vi "Synthetic_Jet_Measurement.vi"() -> (5 "Plug in titles":string[](array[string]), 7 "Plug in values":string[](array[string]))   [LabVIEW 2011]
uses:
  Controls/SJ_Channels.ctl
  Controls/SJ_Data_Cluster.ctl
  <vilib>/Analysis/2dsp.llb/Integral Method.ctl
  Globals/Meas_global.vi
  Globals/Plug_in_data_global.vi
  <vilib>/Analysis/5stat.llb/RMS (DBL).vi
  <vilib>/Analysis/8numeric.llb/1D Numeric Integration.vi
  Utilities/Get_Circ_Area.vi
  <vilib>/Analysis/baseanly.llb/Quick Scale 1D.vi
  <vilib>/Analysis/1siggen.llb/Ramp Pattern by Samples.vi
  <vilib>/Analysis/NI_AALBase.lvlib
  <vilib>/Analysis/NI_AALPro.lvlib
panel:
  out "Jet ID":string="A"
  out "Disc ID":i32
  out "RMS Power 2 _W_":dbl
  out "RMS Input Voltage _V_":dbl format="%0.2f"
  out "Jet Efficiency":dbl
  out "Int Power _W_":dbl
  out "Phase Average?":bool
  out "Samps per cyle":i32
  out "Formation Criteria":dbl
  out "Jet Formation":bool
  out "Strouhal Number":dbl
  out "Stokes Number":dbl
  out "nu":dbl=1.55e-05
  out "Omega":dbl=1200.0
  out "Reynolds Number":dbl
  out "Charicteristic Velocity m_s":dbl
  out "Stroke Length _m_":dbl
  out "DL:Frequency":dbl=2.802671520827615
  out "Cavity:Helmholtz:Hz":dbl=428.16291209383184
  out "DL:Radius":dbl
  out "DL:Streamwise:Position":dbl=5.0
  out "LEM Velocity _ms_":dbl[](array[numeric])=[3.7049856348371377, 3.4607988115264297, 3.0653584733968287, 2.5359472607578692, 1.895702983998723, 1.1726073902466658, 0.3982632267462864, -0.3934869508418966, -1.1680398605184126, -1.8915438234131698, -2.5323782445904723, -3.062535584780142, -3.458845424238726, -3.7039871212762807, -3.787246807411894, -3.7049856348371377, -3.4607988115264297, -3.0653584733968295, -2.5359472607578692, -1.8957029839987247, -1.172607390246666, -0.3982632267462887, 0.3934869508418962, 1.1680398605184101, 1.8915438234131694, 2.53237824459047, 3.0625355847801417, 3.4588454242387248, 3.7039871212762803, 3.7872468074118935]
  out "LEM Max Velocity _ms_":dbl=3.7872475686779676
  out "LEM Phase Velocity _deg_":dbl=-258.0363282123533
  out "Phase Power _deg_":dbl=-1216.295394809798
  out "Phase Current _deg_":dbl=114.2968039724566
  out "RV Phase Pressure _deg_":dbl
  out "Phase Pressure _deg_":dbl=-169.14507601114087
  out "Phase Displ _deg_":dbl=-40.709415815185025
  out "Phase Velocity _deg_":dbl=373.1272896341652
  out "Phase Input Voltage _deg_":dbl=8.606071626556414
  out "Phase Angle _deg_":dbl[](array[numeric])=[0.0, 12.0, 24.0, 36.0, 48.0, 60.0, 72.0, 84.0, 96.0, 108.0, 120.0, 132.0, 144.0, 156.0, 168.0, 180.0, 192.0, 204.0, 216.0, 228.0, 240.0, 252.0, 264.0, 276.0, 288.0, 300.0, 312.0, 324.0, 336.0, 348.0]
  out "Max Power _W_":dbl=0.09567394666235574 format="%0.2f"
  out "Amplitude (V)":dbl=70.0
  out "Frequency (Hz)":dbl=1200.0
  out "AS Freq":dbl=36036.04
  out "Output Data Names":string[](array[string])=["Max Pressure _Pa_", "Max Velocity m_s", "Max Current _A_", "Max Displacement _m_", "Phase Displ _deg_", "Phase Pressure _deg_", "Phase Velocity _deg_", "Phase Current _deg_", "Phase Input Voltage _deg_", "LEM Max Velocity _ms_", "LEM Phase Velocity _deg_"]
  out "Current _A_":dbl[](array[numeric])=[0.007871578951352444, 0.008266417140890889, 0.00849968074403876, 0.008455354076272185, 0.007734598407207069, 0.006567672714377243, 0.00502412226480415, 0.003160545427498193, 0.0011561900642313688, -0.0008322812950871137, -0.0026496409136783387, -0.004250177970402979, -0.0056599044207173484, -0.006974613805967722, -0.007544462997563997, -0.008243629249997945, -0.008448348909812501, -0.008596065082556333, -0.008270248882544743, -0.007591372292965107, -0.0065346555924612445, -0.005182607825984795, -0.003607407527949277, -0.0016626720392260718, 0.00036386353784322137, 0.0021437834956932957, 0.003704399543557329, 0.005128068807114345, 0.006438338773620389, 0.007353635511234548]
  out "Power_W_":dbl[](array[numeric])=[-0.043363451952469156, -0.1045787042911587, -0.16349661489678932, -0.21135096948039916, -0.2294893577920496, -0.21702510361561647, -0.17587031608696657, -0.11191242161210375, -0.03966959410717387, 0.026383849953920794, 0.07342545396353153, 0.09567394666235574, 0.0925358489049179, 0.06622858320017053, 0.01657193795313242, -0.042740863570043953, -0.10421979243576313, -0.16261661392816973, -0.2041915474460092, -0.22315321729709184, -0.2143088761872366, -0.18014115682356102, -0.12703551569073906, -0.05674338994484436, 0.011476164341731257, 0.059131235834024416, 0.08299512964242624, 0.08340916969883025, 0.06053396412209597, 0.01568890358261011]
  out "RV Pressure _V_":dbl[](array[numeric])=[-14.369666524328046, -57.77058962565634, -87.07652966541758, -117.51006835010423, -142.3114261743131, -158.09199483911908, -155.83679754926837, -151.8902022920296, -142.3114261743131, -120.32906496241762, -88.20412831034297, -49.31359978871612, -12.114469234477319, 29.02544421285115, 67.35217341201532, 101.7323073539407, 128.78305010385122, 147.3826153809706, 157.5310031852989, 162.59938472331393, 149.63781267082135, 136.11244129586606, 102.29610667640338, 72.99016663664214, 42.55081558780641, -5.354689729074237, -48.18600114379076, -84.25753305310417, -116.38246970517886, -138.36483091707433, -158.65579416158175, -165.41557366698484, -160.34719212896982, -149.0712056797162, -122.58426225226835, -92.71452289004439, -56.642990980730964, -17.188663136641456, 24.515049633149694, 61.15038086492581, 97.22191277423924, 132.1658460386273, 151.3292106382094, 160.34418743346322, 160.34418743346322, 155.27580589544817, 136.67624061832876, 106.80650125610484, 74.67575223988108, 33.5358387925526, -1.9718937942981463, -42.553820283313044, -85.38513169802953, -116.38246970517886, -141.74762685185044, -159.78339280650712, -164.28797502205947, -162.03859009635784, -141.18382752938774, -123.71186089719372, -94.40592085743245, -59.46198759304437, -20.007659748954865, 21.70186538498539, 58.3313842526124, 92.14771887207513, 124.27846788829885, 149.63781267082135, 160.34418743346322, 156.9672038628362, 155.27580589544817, 141.75043452049292, 110.18348482673184, 77.49474885219449, 41.987016265343726, 0.2833034955525799, -41.42622163838768, -76.37015490277572, -109.62269019977577, -131.59923904752216, -159.21959348404445, -167.67077095683558, -160.9109914514325, -151.8902022920296, -125.96705818704444, -102.29329900776088, -63.96656980859674, -33.53303112391013, 16.627671482821253, 53.82680203706004, 93.27531751700047, 122.58706992091082, 148.51021402589598, 158.65860183022428, 155.27580589544817, 156.9672038628362, 142.30842147880648, 120.3318726310601, 80.31374546450789, 48.18880881243323, 10.425878935731753, -34.6606297688355, -76.37015490277572, -108.49509155485042, -133.85443633737287, -151.8902022920296, -162.03859009635784, -164.28797502205947, -154.709198904343, -135.54583430476092, -104.54849629761163, -71.85976032307427, -32.96923180144745, 7.0430830009556615, 52.135404069672006, 85.95173868913471, 118.64047466367205, 142.30842147880648, 157.5310031852989, 159.78038811100052, 158.09480250776156, 142.30842147880648, 123.71466856583618, 86.5155380115974, 49.316407457358586, 13.244875548045162, -27.33705094096973, -69.04076371076087, -103.42089765268625, -130.4716404025968, -151.8902022920296, -160.34719212896982, -162.60238941882054, -154.14539958188033, -135.54583430476092, -104.54849629761163, -71.85976032307427, -36.91582705868622, 4.793698075254034, 51.007805424746635, 81.44134410943326, 115.82147805135864, 140.62283587556755, 154.1482072505228, 160.9079867559259, 156.40340454037351, 145.69121741358256, 120.89567195352278, 93.27531751700047, 54.95440068198541]
  out "Displacement _m_":dbl[](array[numeric])=[-2.6563452608725367e-05, -3.3033094590941884e-05, -3.489470009695634e-05, -3.608459414033635e-05, -3.599336290251176e-05, -3.300271431749379e-05, -3.056117109155232e-05, -2.2626856342716373e-05, -1.762170629215838e-05, -1.0755312405507711e-05, -5.5370483534114006e-06, -2.8768068802271785e-07, 4.656075893275746e-06, 8.287603580077764e-06, 1.4940431377787088e-05, 1.9792866303780654e-05, 2.4126214474223672e-05, 2.519431617137013e-05, 2.644560368400959e-05, 2.7208727219429685e-05, 2.372973382223118e-05, 2.04641256790127e-05, 1.719906004067715e-05, 1.3689415117589209e-05, 8.043566800208257e-06, 4.4422385518931854e-06, -1.2338996214552368e-06, -5.841845680176716e-06, -1.1396101089811283e-05, -1.6401251140369278e-05]
  out "Input Voltage _V_":dbl[](array[numeric])=[-5.5088632433799996, -12.651031578584, -19.235618350895997, -24.9961110527, -29.670494279084004, -33.04444558276, -35.005182361704, -35.409211536216006, -34.310616683552006, -31.700640287920002, -27.711473499856005, -22.510574222680006, -16.349366000988, -9.495663135284, -2.196569584672, 5.184714435096, 12.336113665324001, 18.917564300223997, 24.689891482827996, 29.395636083331993, 32.795741589576, 34.758786092276, 35.215182844328, 34.127830748423996, 31.539748142271996, 27.582652797175996, 22.404475723135995, 16.265220463328, 9.402109185388, 2.133489422836]
  out "Pressure _Pa_":dbl[](array[numeric])=[-27.3956675953706, 95.65286233449294, 217.28142105099454, 325.3916285730047, 412.49320713856633, 477.62511872885386, 518.8812420389512, 544.5955786383588, 546.2858417945154, 525.7943338813993, 485.98446016799124, 431.53940396868336, 357.29264741860004, 257.81676584697294, 146.44897730607346, 25.39291194062997, -95.29994862668336, -216.63005998968256, -325.4638615668826, -412.65459893301875, -477.423305725176, -519.6780076017092, -543.7330519967387, -544.6659346048561, -524.568602441649, -487.2326508157636, -435.0203186855821, -361.9795522274816, -267.2741357434412, -152.01151538796677]
  out "Zeros":dbl[](array[numeric])=[1.4978743085562871, 0.2341330189017041, -0.35175473981443495, 0.0022887999999999997, -3.0068544366899315, 2.8293]
  out "Velocity m_s":dbl[](array[numeric])=[-0.006589971422005106, -0.006419643065741468, -0.009111611844261746, -0.006030326884042168, -0.004272653157727323, -0.0068849933436421745, -0.010636233235274354, -0.0035467148583991693, -0.008496862890472292, -0.005357351691532665, -0.007065956289182962, -0.006648911559621155, -0.005058171342073957, -0.008830133605031026, -0.0038751674420970687, -0.005274584307176274, 0.000979796600094568, -0.005616008146962059, -0.00729733372181674, 0.0005036149760482819, -0.004633370846616606, -0.007598533001820504, -0.005354959759266961, -0.003855515705978843, -0.005082756078867318, -0.0008163141834672163, -0.007346968606858383, -0.00413574997102441, -0.00277648312445221, -0.00052352239052674]
  out "Max Current _A_":dbl=0.00849968074403876 format="%e"
  out "RMS Dispacement _m_":dbl=2.25005755896471e-05 format="%0.2f"
  out "RMS Velocity m_s":dbl=0.014914535983039488 format="%0.2f"
  out "RMS Current _A_":dbl=0.006206722435388947 format="%0.2f"
  out "RV RMS Pressure _V_":dbl format="%0.2f"
  out "RMS Pressure _Pa_":dbl=395.7699897259115 format="%0.2f"
  out "RMS Power _W_":dbl=0.13002833315099252 format="%0.2f"
  out "Max Displacement _m_":dbl=2.7208727219429685e-05 format="%e"
  out "Max Pressure _Pa_":dbl=546.2858417945154 format="%0.2f"
  out "RV Max Pressure _V_":dbl format="%0.2f"
  out "Max Velocity m_s":dbl=0.000979796600094568
  out "Current Plot":cluster{dbl[], dbl[]}[](graph)=[{[0.0, 12.0, 24.0, 36.0, 48.0, 60.0, 72.0, 84.0, 96.0, 108.0, 120.0, 132.0, 144.0, 156.0, 168.0, 180.0, 192.0, 204.0, 216.0, 228.0, 240.0, 252.0, 264.0, 276.0, 288.0, 300.0, 312.0, 324.0, 336.0, 348.0], [-0.15557712257291065, -0.35728080433659803, -0.5432376920119246, -0.705921142218441, -0.8379315153272326, -0.9332160799164545, -0.9885897155857659, -1.0, -0.9689743203815658, -0.8952653536353687, -0.7826063416157439, -0.6357265029653804, -0.4617263500562873, -0.2681692905127802, -0.06203384626131485, 0.1464227586596542, 0.34838713233438734, 0.5342554516040381, 0.697273122209331, 0.8301691793748806, 0.926192371045399, 0.9816311796924717, 0.9945203893712923, 0.9638122191316959, 0.8907215601232357, 0.7789682853842954, 0.632730149899583, 0.45934997583022086, 0.26552721106968635, 0.060252384345070756]}, {[0.0, 12.0, 24.0, 36.0, 48.0, 60.0, 72.0, 84.0, 96.0, 108.0, 120.0, 132.0, 144.0, 156.0, 168.0, 180.0, 192.0, 204.0, 216.0, 228.0, 240.0, 252.0, 264.0, 276.0, 288.0, 300.0, 312.0, 324.0, 336.0, 348.0], [0.915718863893427, 0.9616512975995976, 0.9887873884629885, 0.9836307653638304, 0.8997836024883751, 0.7640324556993839, 0.5844676856855597, 0.36767351074525567, 0.13450224644966696, -0.09682119517406056, -0.3082388148799797, -0.49443296782707047, -0.6584296845544803, -0.8113728478069623, -0.8776647134598465, -0.9590003298982027, -0.9828158382556238, -1.0, -0.962097052909388, -0.8831217795651628, -0.7601914980520298, -0.6029046751288172, -0.41965800552972216, -0.19342245821289428, 0.04232908131205239, 0.24939125926856856, 0.4309413095387709, 0.5965600257634787, 0.7489867412341333, 0.855465313560387]}]
  in  "Menu Ring":u16(ring) items=["Max Pressure _Pa_", "RMS Pressure _Pa_", "Phase Pressure _deg_", "Max Current _A_", "RMS Current _A_", "Phase Current _deg_", "Max Power _W_", "RMS Power _W_", "RMS Power 2 _W_", "Int Power _W_", "Phase Power _deg_"]
  out "Pressure v Frequency":cluster{dbl[], dbl[]}(graph)
  out "Pressure Plot":cluster{dbl[], dbl[]}[](graph)=[{[0.0, 12.0, 24.0, 36.0, 48.0, 60.0, 72.0, 84.0, 96.0, 108.0, 120.0, 132.0, 144.0, 156.0, 168.0, 180.0, 192.0, 204.0, 216.0, 228.0, 240.0, 252.0, 264.0, 276.0, 288.0, 300.0, 312.0, 324.0, 336.0, 348.0], [-0.15557712257291065, -0.35728080433659803, -0.5432376920119246, -0.705921142218441, -0.8379315153272326, -0.9332160799164545, -0.9885897155857659, -1.0, -0.9689743203815658, -0.8952653536353687, -0.7826063416157439, -0.6357265029653804, -0.4617263500562873, -0.2681692905127802, -0.06203384626131485, 0.1464227586596542, 0.34838713233438734, 0.5342554516040381, 0.697273122209331, 0.8301691793748806, 0.926192371045399, 0.9816311796924717, 0.9945203893712923, 0.9638122191316959, 0.8907215601232357, 0.7789682853842954, 0.632730149899583, 0.45934997583022086, 0.26552721106968635, 0.060252384345070756]}, {[0.0, 12.0, 24.0, 36.0, 48.0, 60.0, 72.0, 84.0, 96.0, 108.0, 120.0, 132.0, 144.0, 156.0, 168.0, 180.0, 192.0, 204.0, 216.0, 228.0, 240.0, 252.0, 264.0, 276.0, 288.0, 300.0, 312.0, 324.0, 336.0, 348.0], [-0.05014896140338823, 0.1750967259562854, 0.39774309423293575, 0.5956435325215701, 0.7550867615085017, 0.8743135592895557, 0.9498346878887768, 0.9969058997564276, 1.0, 0.9624894032658751, 0.8896156974736197, 0.7899516534258018, 0.6540397353973438, 0.47194480640402603, 0.2680812243366908, 0.0464828300459258, -0.17445070206035157, -0.39655074947222896, -0.5957757581594167, -0.7553821962097238, -0.87394413180629, -0.9512932019153176, -0.9953270072140422, -0.9970346894139926, -0.9602456485390019, -0.8919005647578826, -0.7963236192550169, -0.6626193185574809, -0.4892569334498257, -0.2782636922981901]}]
  out "Displacement Plot":cluster{dbl[], dbl[]}[](graph)=[{[0.0, 12.0, 24.0, 36.0, 48.0, 60.0, 72.0, 84.0, 96.0, 108.0, 120.0, 132.0, 144.0, 156.0, 168.0, 180.0, 192.0, 204.0, 216.0, 228.0, 240.0, 252.0, 264.0, 276.0, 288.0, 300.0, 312.0, 324.0, 336.0, 348.0], [-0.15557712257291065, -0.35728080433659803, -0.5432376920119246, -0.705921142218441, -0.8379315153272326, -0.9332160799164545, -0.9885897155857659, -1.0, -0.9689743203815658, -0.8952653536353687, -0.7826063416157439, -0.6357265029653804, -0.4617263500562873, -0.2681692905127802, -0.06203384626131485, 0.1464227586596542, 0.34838713233438734, 0.5342554516040381, 0.697273122209331, 0.8301691793748806, 0.926192371045399, 0.9816311796924717, 0.9945203893712923, 0.9638122191316959, 0.8907215601232357, 0.7789682853842954, 0.632730149899583, 0.45934997583022086, 0.26552721106968635, 0.060252384345070756]}, {[0.0, 12.0, 24.0, 36.0, 48.0, 60.0, 72.0, 84.0, 96.0, 108.0, 120.0, 132.0, 144.0, 156.0, 168.0, 180.0, 192.0, 204.0, 216.0, 228.0, 240.0, 252.0, 264.0, 276.0, 288.0, 300.0, 312.0, 324.0, 336.0, 348.0], [-0.7361438653132033, -0.9154348379941063, -0.9670248738630008, -1.0, -0.997471739948916, -0.9145929198799676, -0.8469312685822951, -0.6270503211070746, -0.48834431180314575, -0.2980582894650082, -0.15344632481876624, -0.00797239638899362, 0.12903223672595104, 0.2296715198692966, 0.4140390583217413, 0.5485129256769343, 0.668601519540294, 0.6982014560947281, 0.7328779584207091, 0.7540261396210363, 0.6576139870090829, 0.5671153068654675, 0.47663166097388826, 0.3793700731217815, 0.22290861216080401, 0.12310623571424707, -0.03419463765219268, -0.16189306875552578, -0.3158162468307329, -0.45452225613466185]}]
  out "Velocity Plot":cluster{dbl[], dbl[]}[](graph)=[{[0.0, 12.0, 24.0, 36.0, 48.0, 60.0, 72.0, 84.0, 96.0, 108.0, 120.0, 132.0, 144.0, 156.0, 168.0, 180.0, 192.0, 204.0, 216.0, 228.0, 240.0, 252.0, 264.0, 276.0, 288.0, 300.0, 312.0, 324.0, 336.0, 348.0], [-0.15557712257291065, -0.35728080433659803, -0.5432376920119246, -0.705921142218441, -0.8379315153272326, -0.9332160799164545, -0.9885897155857659, -1.0, -0.9689743203815658, -0.8952653536353687, -0.7826063416157439, -0.6357265029653804, -0.4617263500562873, -0.2681692905127802, -0.06203384626131485, 0.1464227586596542, 0.34838713233438734, 0.5342554516040381, 0.697273122209331, 0.8301691793748806, 0.926192371045399, 0.9816311796924717, 0.9945203893712923, 0.9638122191316959, 0.8907215601232357, 0.7789682853842954, 0.632730149899583, 0.45934997583022086, 0.26552721106968635, 0.060252384345070756]}, {[0.0, 12.0, 24.0, 36.0, 48.0, 60.0, 72.0, 84.0, 96.0, 108.0, 120.0, 132.0, 144.0, 156.0, 168.0, 180.0, 192.0, 204.0, 216.0, 228.0, 240.0, 252.0, 264.0, 276.0, 288.0, 300.0, 312.0, 324.0, 336.0, 348.0], [-0.0017400427690923374, -0.0016950685794170583, -0.002405866928563968, -0.0015922719565676093, -0.001128168660507009, -0.0018179415532591603, -0.002808434141249664, -0.0009364889690996669, -0.002243546122698781, -0.0014145768585897204, -0.0018657237429983216, -0.001755605561963586, -0.0013355800662831847, -0.0023315442732039188, -0.0010232149208002786, -0.001392722622896813, 0.00025870946624789303, -0.0014828735576385352, -0.0019268175782828233, 0.00013297653986074366, -0.0012234140213805954, -0.002006347457194939, -0.0014139452830977239, -0.0010180259967302217, -0.001342071519849202, -0.00021554290622666447, -0.0019399233745421283, -0.001092020188103525, -0.0007331138596561618, -0.00013823297428152076]}, {[0.0, 12.0, 24.0, 36.0, 48.0, 60.0, 72.0, 84.0, 96.0, 108.0, 120.0, 132.0, 144.0, 156.0, 168.0, 180.0, 192.0, 204.0, 216.0, 228.0, 240.0, 252.0, 264.0, 276.0, 288.0, 300.0, 312.0, 324.0, 336.0, 348.0], [0.9782794265180274, 0.9138033477917035, 0.8093896778519208, 0.6696017951074252, 0.5005491008108334, 0.3096200089077361, 0.10515903689372944, -0.10389788964157722, -0.3084139798421589, -0.49945089918916635, -0.6686594176102914, -0.8086443108979737, -0.9132875674934984, -0.9780157749495838, -1.0, -0.9782794265180274, -0.9138033477917035, -0.8093896778519211, -0.6696017951074252, -0.5005491008108338, -0.30962000890773617, -0.10515903689373006, 0.10389788964157712, 0.3084139798421583, 0.4994508991891662, 0.6686594176102908, 0.8086443108979736, 0.9132875674934979, 0.9780157749495837, 0.9999999999999999]}]
  out "Amplitude String":string="3.5000"
  out "Frequency String":string="1200"
  # "You Must have selected the \"Save Data\" option on the \nMeasurement Program for this vi to work correctly"
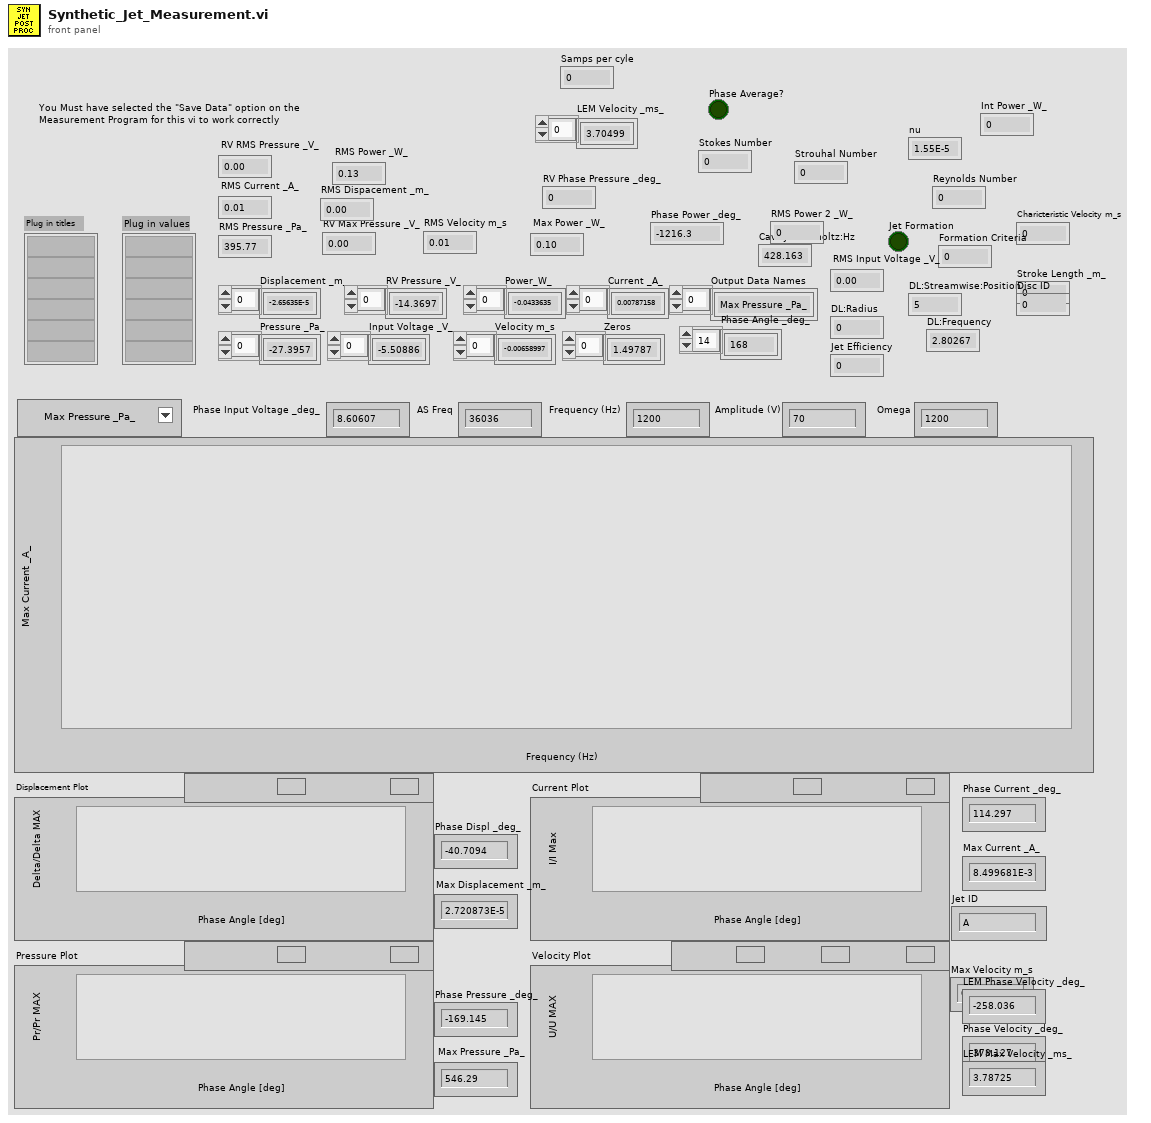
[diagram p1: front panel]
types:
  T1 = typedef "SJ_Channels.ctl" = string[]
  T2 = typedef "Analysis_info_cluster.ctl" = cluster{"Colour":u32, "Inst type":T3, "Inst name":string, "Symbol":string, "Code name":string, "Extra Info":string, "Inst Array":T4, "Extra Titles":string[], "Extra Values":string[], "Eng Values":dbl[], "Time (ms)":dbl[], "Voltage":dbl[], "U":dbl, "u^2":dbl, "u^3":dbl, "u^4":dbl, "Skew_u":dbl, "Kurt_u":dbl, "Sd Error in Mean":dbl, "% u'/U":dbl, "X":dbl, "Y":dbl, "Z":dbl, "Spectra":T5, "Autocorrelation":T5, "Timescale integral to 25%":dbl, "Sd Error in Variance":dbl, "Calib File":path, "Calib Constants":dbl[], "Histogram":T5, "Output Position":bool, "Full Stats":bool, "Weighting":dbl[], "Av Sampling Rate":dbl, "Av No of Samples":dbl, "Total Meas Time (s)":dbl}
  T3 = typedef "Inst_type.ctl" = enum16{"Propeller anemometer", "Raw voltage", "Pressure Transducer", "Pitot-static tube", "Preston tube", "Hot wire", "Cross wire 1", "Cross wire 2", "Generic Linear", "Generic Polynomial", "Generic BackPoly", "Fast FID", "Thermocouple", "Cold wire", "Pulsed Wire", "LDA Vel", "LDA Tran time", "LDA Arr time"}
  T4 = typedef "Instrument_Array.ctl" = enum16{"PWA", "LDA", "Analogue"}
  T5 = typedef "XY_Plot_Cluster.ctl" = cluster{"First Name":string, "Second Name":string, "X axis name":string, "Y axis name":string, "X array":dbl[], "Y array":dbl[]}
  T6 = typedef "Post_Process.ctl" = enum16{"Take New Data", "Post Process Raw Data File"}
  T7 = typedef "SJ_Data_Cluster.ctl" = cluster{"Do":dbl, "Dc":dbl, "Ho":dbl, "Hc":dbl, "K":dbl, "beta":dbl, "Vc":dbl, "Vo":dbl}
  T8 = cluster{"R":dbl, "Mair":dbl, "T":dbl, "Patmos":dbl, "gamma":dbl}
  T9 = typedef "NI_AALPro.lvlib/Integral Method.ctl" = i32
  T10 = cluster{"Ramp Pattern":dbl[], "Y[i]=X[i]/Max|X|":dbl[]}
  T11 = cluster{"Ramp Pattern":dbl[], "Y[i]=X[i]/Max|X|":dbl[]}[]
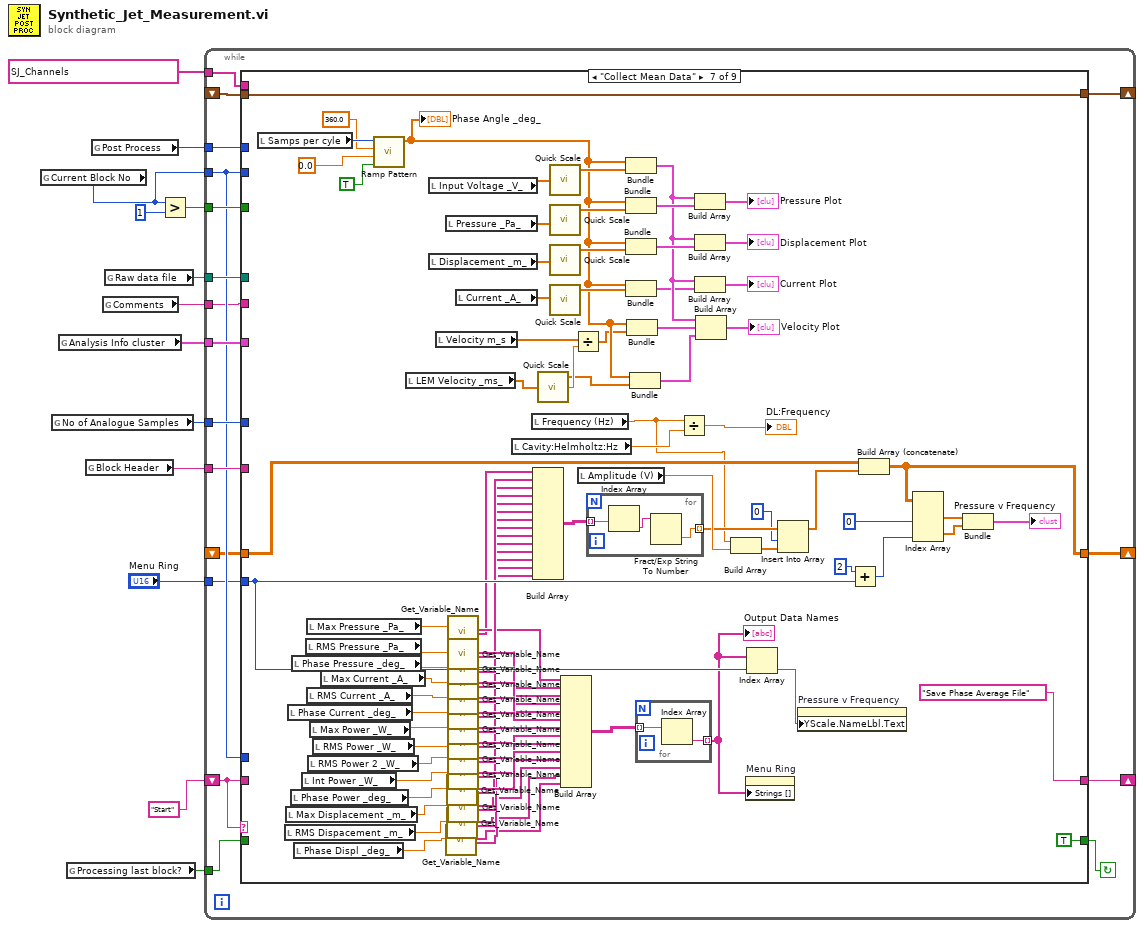
[diagram p0: block diagram]
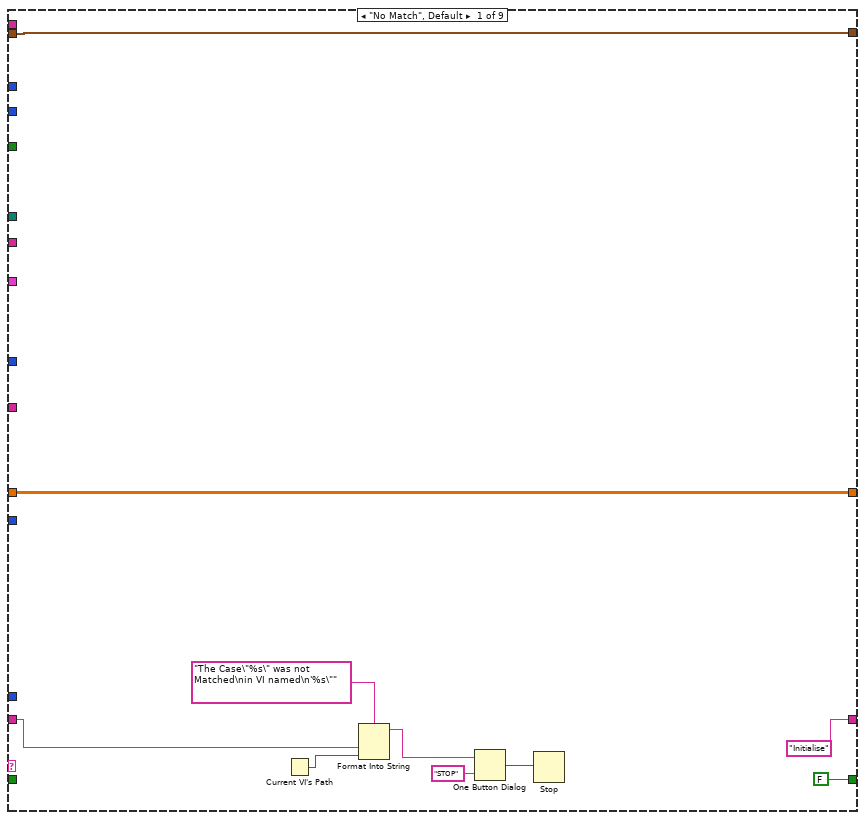
[diagram p2: hidden frame]
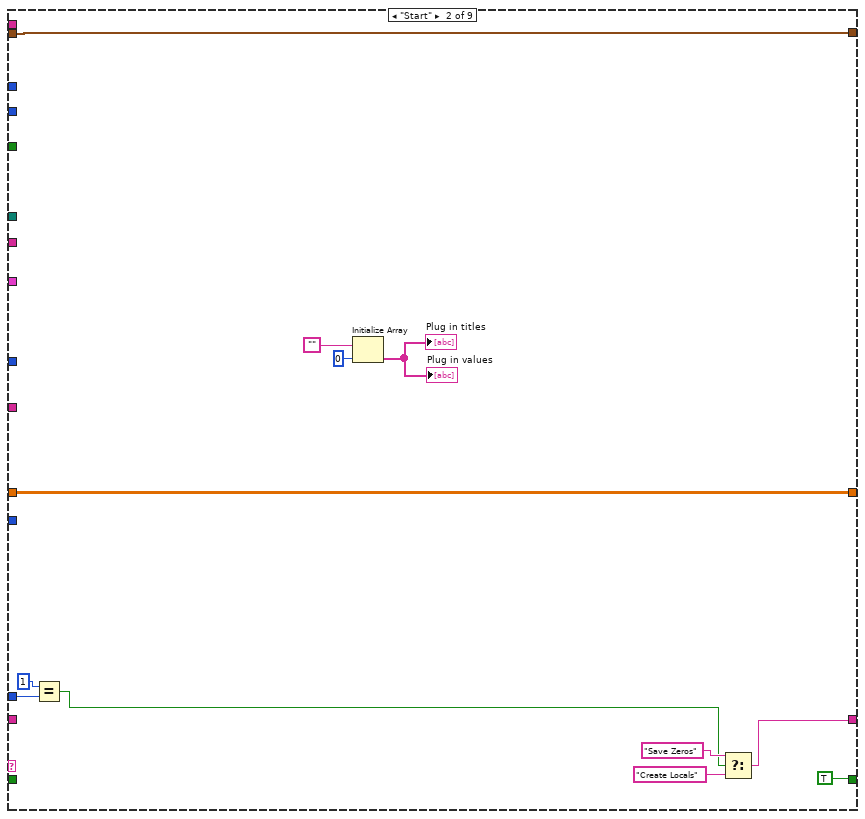
[diagram p3: hidden frame]
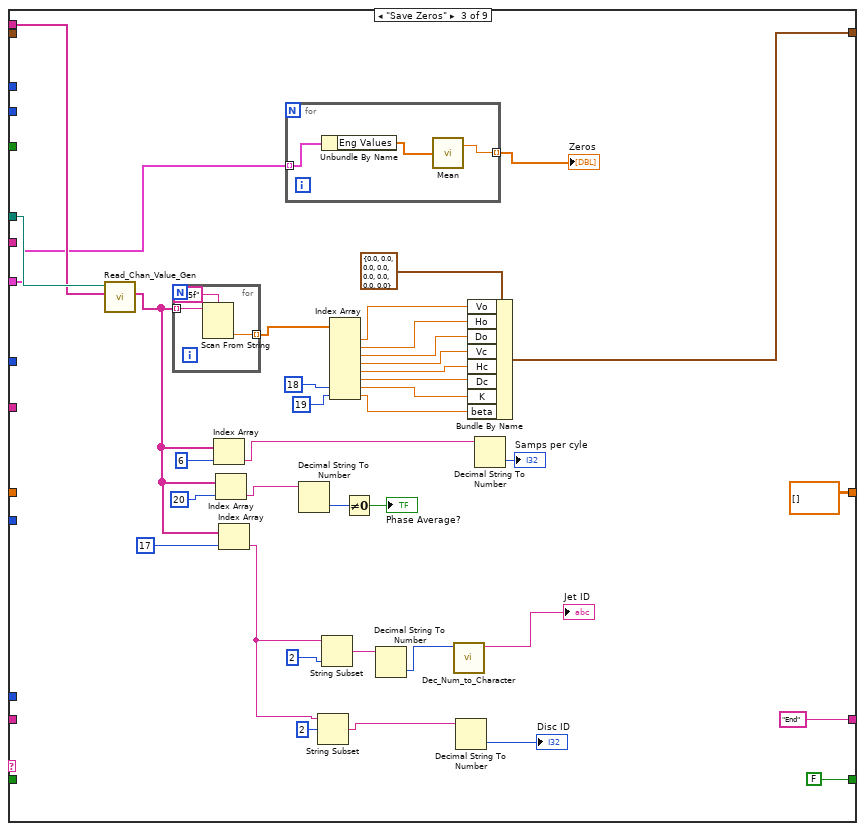
[diagram p4: hidden frame]
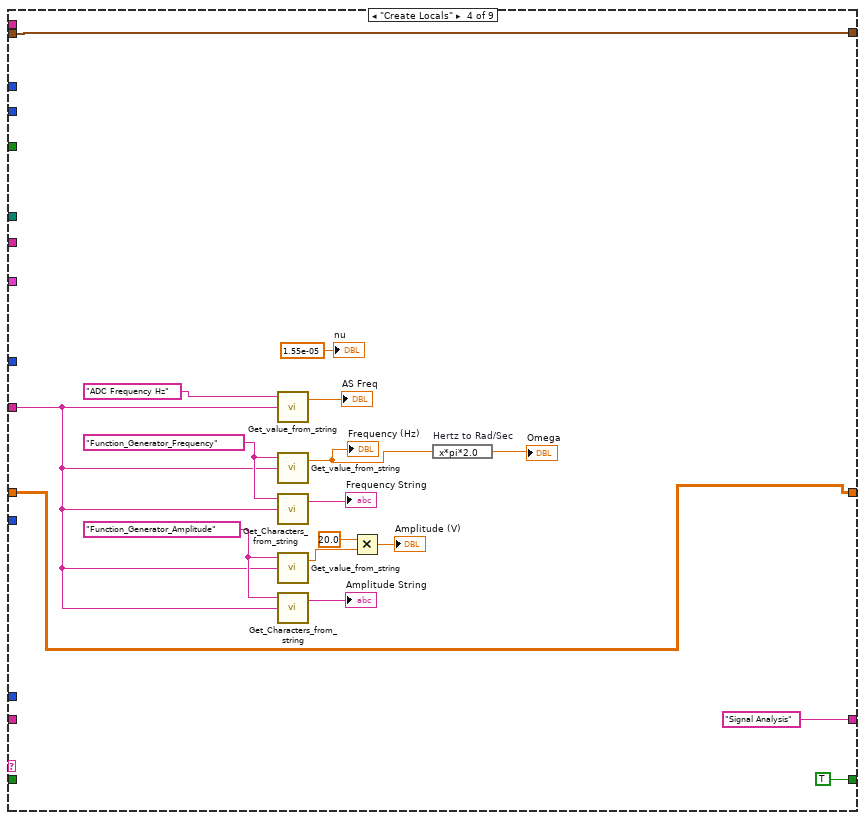
[diagram p5: hidden frame]
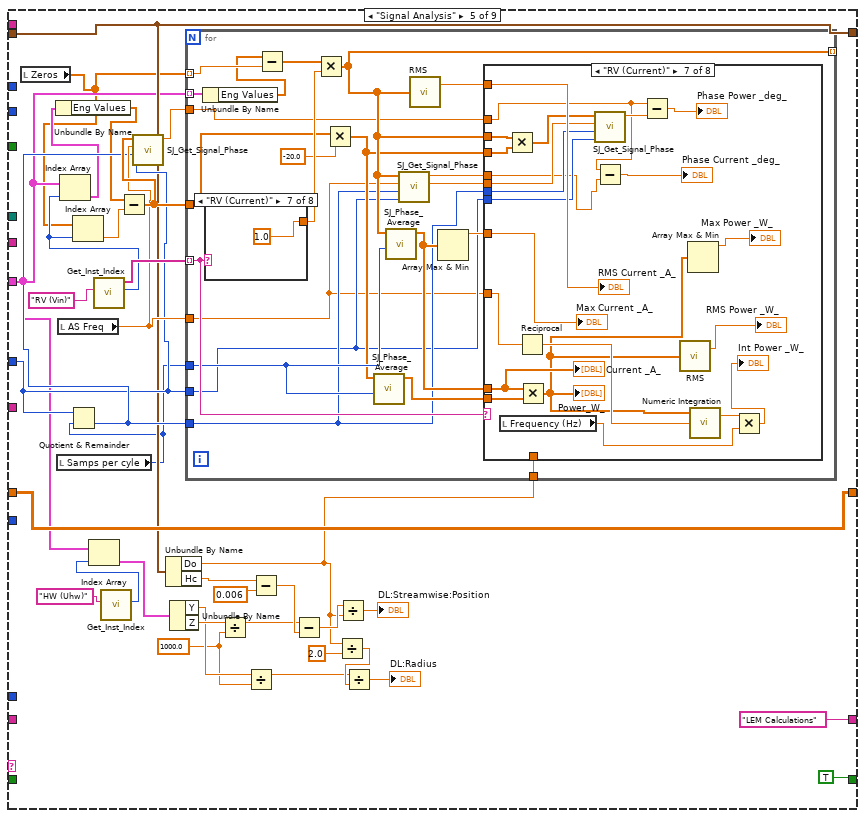
[diagram p6: hidden frame]
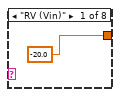
[diagram p7: hidden frame]
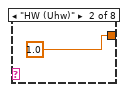
[diagram p8: hidden frame]
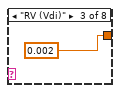
[diagram p9: hidden frame]
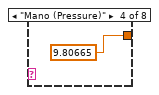
[diagram p10: hidden frame]
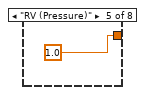
[diagram p11: hidden frame]
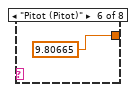
[diagram p12: hidden frame]
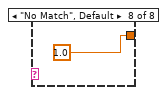
[diagram p13: hidden frame]
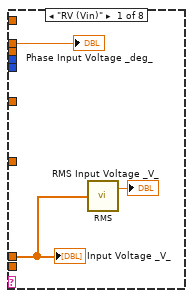
[diagram p14: hidden frame]
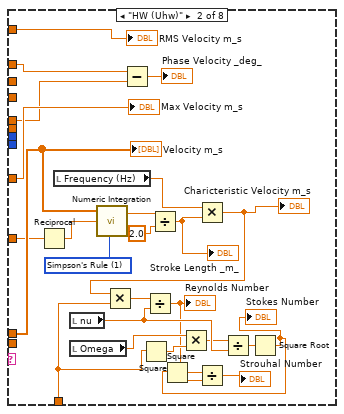
[diagram p15: hidden frame]
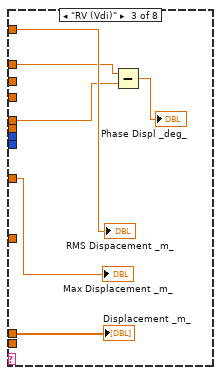
[diagram p16: hidden frame]
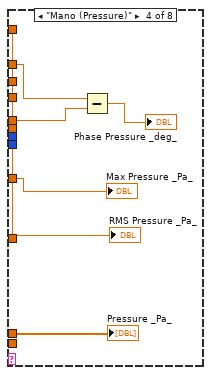
[diagram p17: hidden frame]
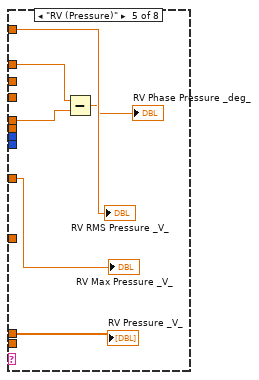
[diagram p18: hidden frame]
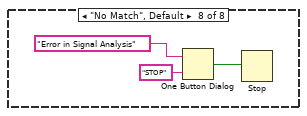
[diagram p20: hidden frame]
diagram:
  n1 = global read "Meas_global.vi" "Current Block No"() -> (w9:i32)
  n2 = global read "Meas_global.vi" "No of Analogue Samples"() -> (w6:i32)
  n3 = global read "Meas_global.vi" "Analysis Info cluster"() -> (w8:T2[])
  n4 = global read "Meas_global.vi" "Processing last block?"() -> (w5:bool)
  n5 = global read "Plug_in_data_global.vi" "Block Header"() -> (w7:string)
  n6 = global read "Meas_global.vi" "Post Process"() -> (w2:T6)
  n7 = global read "Meas_global.vi" "Comments"() -> (w4:string)
  n8 = global read "Meas_global.vi" "Raw data file"() -> (w12:path)
  n9 = Greater?(x=w9, y=1) -> (0:w10:bool)
  n10 = while {
    shift-left: "Start" -> [w31]
    shift-right: [w23] -> _
    tunnel: w12 -> [w30]
    tunnel: w10 -> [w29]
    tunnel: w9 -> [w24]
    tunnel: w8 -> [w28]
    tunnel: w7 -> [w27]
    tunnel: w6 -> [w26]
    tunnel: w5 -> [w25]
    shift-right: [w21] -> _
    shift-left: _ -> [w20]
    tunnel: w4 -> [w19]
    tunnel: "Menu Ring" -> [w18]
    tunnel: w2 -> [w17]
    shift-right: [w15] -> _
    shift-left: _ -> [w16]
    tunnel: T1 ["Synthetic_Jet:Orifice:Volume", "Synthetic_Jet:Orifice:Height", "Synthetic_Jet:Orifice:Diameter", "Synthetic_Jet:Cavity:Volume", "Synthetic_Jet:Cavity:Height", "Synthetic_Jet:Cavity:Diameter", "Synthetic_Jet:Samples:Per_Cycle", "Synthetic_Jet:Dwell:Time", "Synthetic_Jet:Minimum:Frequency", "Synthetic_Jet:Maximum:Frequency", "Synthetic_Jet:Minimum:Amplitude", "Synthetic_Jet:Maximum:Amplitude", "Synthetic_Jet:Amplitude:Delta", "Synthetic_Jet:Frequency:Delta", "Synthetic_Jet:Calibration:Velocity", "Synthetic_Jet:Calibration:Type", "Synthetic_Jet:Calibration:No_Of_Gens", "Synthetic_Jet:Identification:Number", "Synthetic_Jet:LEM_Pressure:Coefficient", "Synthetic_Jet:LEM_Added_Mass:Coefficient", "Synthetic_Jet:Phase:Average?", "Synthetic_Jet:Optimisation:Coefficient"] ("Synthetic Jet Specific Channels") -> [w14]
    stop <- w22 continue-if-true
    n11 = case shown="\"Collect Mean Data\"" w31 {
      tunnel: w31 -> [w37 _ _ _ _ _ _ _ _]
      tunnel: w30 -> [_ _ w84 _ _ w271 _ w468 w516]
      tunnel: w29 -> [_ _ _ _ _ _ _ _ _]
      tunnel: w24 -> [_ _ _ _ _ _ _ _ _]
      tunnel: w28 -> [_ _ w54 _ w116 _ _ _ _]
      tunnel: w27 -> [_ _ _ w108 _ _ _ _ _]
      tunnel: w26 -> [_ _ _ _ w138 _ _ _ _]
      tunnel: w25 -> [_ _ _ _ _ _ _ w395 _]
      tunnel: w24 -> [_ w50 _ _ _ _ _ _ _]
      tunnel: ["Initialise" w46 "End" ("t") "Signal Analysis" "LEM Calculations" "Collect Mean Data" "Save Phase Average File" "Save Mean Data" ("t") "End"] -> w23
      tunnel: [FALSE TRUE FALSE TRUE TRUE TRUE ("Processing last block?") TRUE ("Processing last block?") w395 FALSE ("Processing last block?")] -> w22
      tunnel: [w33 w44 dbl[][] [] w105 w144 w293 w379 w408 w558] -> w21
      tunnel: w20 -> [w33 w44 _ w105 w144 w293 w380 w408 w558]
      tunnel: w19 -> [_ _ _ _ _ _ _ w410 w532]
      tunnel: w18 -> [_ _ _ _ _ _ w354 _ _]
      tunnel: w17 -> [_ _ _ _ _ _ _ _ _]
      tunnel: w16 -> [w32 w42 _ w97 w133 w260 w316 w422 w557]
      tunnel: [w32 w42 w85 w97 w133 w260 w316 w422 w557] -> w15
      tunnel: w14 -> [_ _ w83 _ _ _ _ _ _]
      frame "No Match", Default {
        n12 = Current VI's Path() -> (path=w36:path)
        n13 = Format Into String(format string="The Case\"%s\" was not Matched\nin VI named\n'%s\"" ("Format String"), w37, w36) -> (resulting string=w40:string)  [unwired: 2 in, 1 out]
        n14 = One Button Dialog(message=w40, button name ("OK")="STOP") -> (true=w38:bool)
        n15 = Stop(stop? (T)=w38) -> ()
      }
      frame "Start" {
        n16 = Equal?(x=1, y=w50) -> (x = y?=w43:bool)
        n17 = Initialize Array("", 0) -> (→"Plug in values" →"Plug in titles":string[])
        n18 = Select(t="Save Zeros", s=w43, f="Create Locals") -> (s? t:f=w46:string)
      }
      frame "Save Zeros" {
        (unwired) FALSE ("Processing last block?")
        (unwired) "End" ("t")
        (unwired) "End" ("t")
        (unwired) FALSE ("Processing last block?")
        n19 = call "Read_Chan_Value_Gen.vi"("Desired Ch Names"=w83, "Raw data file"=w84) -> ("Values"=w63:string[])  [unwired: 9 in]
        n20 = for {
          tunnel: w63 -> [w93] mode=indexing
          tunnel: [w91] -> w72 mode=indexing
          n21 = Scan From String(format string="%5f", input string=w93) -> (output 1=w91:dbl)  [unwired: 3 in, 3 out]
        }
        n22 = Index Array(array=w63, index=6) -> (element=w70:string)
        n23 = Index Array(array=w63, index=20) -> (element=w67:string)
        n24 = Index Array(array=w63, index=17) -> (element=w55:string)
        n25 = for {
          tunnel: [w96] -> w89 mode=indexing
          tunnel: w54 -> [w95] mode=indexing
          n26 = Unbundle By Name(w95) -> ("Eng Values"=w94:dbl[])
          n27 = call <vilib>:"Mean.vi"("X"=w94) -> ("mean"=w96:dbl)  [unwired: 1 out]
        }
        "Zeros" <- w89
        n28 = Decimal String To Number(string=w67) -> (number=w66:i32)  [unwired: 2 in, 1 out]
        n29 = String Subset(string=w55, offset (0)=2) -> (substring=w58:string)  [unwired: 1 in]
        n30 = String Subset(string=w55, length (rest)=2 ("length (rest)")) -> (substring=w59:string)  [unwired: 1 in]
        n31 = Index Array(array=w72, index #7=18 ("index"), index #8=19 ("index")) -> (element #1=w82:dbl, element #2=w81:dbl, element #3=w80:dbl, element #4=w79:dbl, element #5=w78:dbl, element #6=w77:dbl, element #7=w74:dbl, element #8=w73:dbl)  [unwired: 6 in]
        n32 = Not Equal To 0?(x=w66) -> (x != 0?=→"Phase Average?":bool)
        n33 = Decimal String To Number(string=w59) -> (number=w57:i32)  [unwired: 2 in, 1 out]
        n34 = call "Dec_Num_to_Character.vi"("Decimal Number"=w57) -> ("Output String"=→"Jet ID":string)  [unwired: 10 in]
        n35 = Decimal String To Number(string=w58) -> (number=→"Disc ID":i32)  [unwired: 2 in, 1 out]
        n36 = Bundle By Name(cluster=T7 {"Do"=0.0, "Dc"=0.0, "Ho"=0.0, "Hc"=0.0, "K"=0.0, "beta"=0.0, "Vc"=0.0, "Vo"=0.0} ("SJ_Data_Cluster"), "Vo"=w82, "Ho"=w81, "Do"=w80, "Vc"=w79, "Hc"=w78, "Dc"=w77, "K"=w74, "beta"=w73) -> (w85:T7)
        n37 = Decimal String To Number(string=w70) -> (number=→"Samps per cyle":i32)  [unwired: 2 in, 1 out]
      }
      frame "Create Locals" {
        w110 = "Function_Generator_Amplitude" ("Variable name")
        w111 = "Function_Generator_Frequency" ("Variable name")
        n38 = call "Get_value_from_string.vi"("Input string"=w108, "Variable name"="ADC Frequency Hz") -> ("Value"=→"AS Freq":dbl)  [unwired: 1 in, 1 out]
        n39 = call "Get_value_from_string.vi"("Input string"=w108, "Variable name"=w111) -> ("Value"=w100:dbl)  [unwired: 1 in, 1 out]
        "Frequency (Hz)" <- w100
        n40 = call "Get_Characters_from_string.vi"("Input string"=w108, "Variable name"=w111) -> ("Value"=→"Frequency String":string)  [unwired: 1 in, 1 out]
        n41 = call "Get_value_from_string.vi"("Input string"=w108, "Variable name"=w110) -> ("Value"=w103:dbl)  [unwired: 1 in, 1 out]
        n42 = call "Get_Characters_from_string.vi"("Input string"=w108, "Variable name"=w110) -> ("Value"=→"Amplitude String":string)  [unwired: 1 in, 1 out]
        n43 = Multiply(x=20.0, y=w103) -> (x*y=→"Amplitude (V)":dbl)
        n44 = expression code="x*pi*2.0" "Hertz to Rad/Sec"(w100) -> (→"Omega":dbl)
        "nu" <- 1.55e-05 ("y")
      }
      frame "Signal Analysis" {
        w120 = 1000.0 ("y")
        n45 = local read "Zeros"() -> (w115:dbl[])
        n46 = local read "Samps per cyle"() -> (w114:i32)
        n47 = local read "AS Freq"() -> (w140:dbl)
        n48 = Quotient & Remainder(x=w138, y=w114) -> (floor(x/y)=w139:i32)  [unwired: 1 out]
        n49 = call "Get_Inst_Index.vi"("Inst name search"="RV (Vin)" ("element")) -> ("Index of Instance"=w142:i32, "Inst Name Array"=w145:string[])  [unwired: 8 in, 1 out]
        n50 = Index Array(array=w116, index=w142) -> (element=w118:T2)
        n51 = Unbundle By Name(w118) -> ("Eng Values"=w117:dbl[])
        n52 = Index Array(array=w115, index=w142) -> (element=w143:dbl)
        n53 = call "Get_Inst_Index.vi"("Inst name search"="HW (Uhw)" ("element")) -> ("Index of Instance"=w135:i32)  [unwired: 8 in, 2 out]
        n54 = Index Array(array=w116, index=w135) -> (element=w134:T2)
        n55 = Subtract(x=w117, y=w143) -> (x-y=w141:dbl[])
        n56 = call "SJ_Get_Signal_Phase.vi"("No of Analogue Samples"=w138, "Number of Cycles"=w139, "Actual Sampling Frequency"=w140, "Signal"=w141) -> ("Phase Angle"=w137:dbl)  [unwired: 7 in]
        n57 = Unbundle By Name(w133) -> ("Do"=w119:dbl, "Hc"=w132:dbl)
        n58 = Unbundle By Name(w134) -> ("Y"=w124:dbl, "Z"=w129:dbl)
        n59 = for {
          tunnel: w115 -> [w169] mode=indexing
          tunnel: [w158] -> _ mode=indexing
          tunnel: w145 -> [w167] mode=indexing
          tunnel: w114 -> [w160]
          tunnel: w140 -> [w152]
          tunnel: w138 -> [w155]
          tunnel: w139 -> [w156]
          tunnel: w141 -> [w154]
          tunnel: w137 -> [w153]
          tunnel: w119 -> [w151]
          tunnel: w116 -> [w150] mode=indexing
          n60 = Unbundle By Name(w150) -> ("Eng Values"=w149:dbl[])
          n61 = case shown="\"RV (Current)\"" w167 {
            tunnel: [-20.0 1.0 0.002 9.80665 1.0 9.80665 1.0 1.0] -> w165
            frame "RV (Vin)" {
            }
            frame "HW (Uhw)" {
            }
            frame "RV (Vdi)" {
            }
            frame "Mano (Pressure)" {
            }
            frame "RV (Pressure)" {
            }
            frame "Pitot (Pitot)" {
            }
            frame "RV (Current)" {
            }
            frame "No Match", Default {
            }
          }
          n62 = Subtract(x=w149, y=w169) -> (x-y=w168:dbl[])
          n63 = Multiply(x=w168, y=w165) -> (x*y=w158:dbl[])
          n64 = Multiply(x=w154, y=-20.0) -> (x*y=w157:dbl[])
          n65 = call "SJ_Phase_Average.vi"("No. of Bins"=w160, "1D Signal"=w157) -> ("Phase Averaged Signal"=w163:dbl[])  [unwired: 6 in, 3 out]
          n66 = call "SJ_Phase_Average.vi"("No. of Bins"=w160, "1D Signal"=w158) -> ("Phase Averaged Signal"=w162:dbl[])  [unwired: 6 in, 3 out]
          n67 = call "SJ_Get_Signal_Phase.vi"("No of Analogue Samples"=w155, "Number of Cycles"=w156, "Actual Sampling Frequency"=w152, "Signal"=w158) -> ("Phase Angle"=w159:dbl)  [unwired: 7 in]
          n68 = call-poly <vilib>:"RMS.vi"("X"=w158) -> ("rms value"=w166:dbl)  [unwired: 1 out]
          n69 = Array Max & Min(array=w162) -> (max value=w161:dbl)  [unwired: 3 out]
          n70 = case shown="\"RV (Current)\"" w167 {
            tunnel: w162 -> [w179 w200 w211 w217 w223 _ w245 _]
            tunnel: w163 -> [_ _ _ _ _ _ w246 _]
            tunnel: w166 -> [_ w205 w210 w216 w222 _ w243 _]
            tunnel: w161 -> [_ w204 w209 w215 w221 _ w242 _]
            tunnel: w159 -> [w180 w203 w207 w213 w219 _ w232 _]
            tunnel: w158 -> [_ _ _ _ _ _ w240 _]
            tunnel: w157 -> [_ _ _ _ _ _ w239 _]
            tunnel: w152 -> [_ _ _ _ _ _ w237 _]
            tunnel: w156 -> [_ _ _ _ _ _ w236 _]
            tunnel: w155 -> [_ _ _ _ _ _ w235 _]
            tunnel: w153 -> [_ w202 w206 w214 w220 _ w230 _]
            tunnel: w152 -> [_ w198 _ _ _ _ w229 _]
            tunnel: w151 -> [_ w189 _ _ _ _ _ _]
            frame "RV (Vin)" {
              n71 = call-poly <vilib>:"RMS.vi"("X"=w179) -> ("rms value"=→"RMS Input Voltage _V_":dbl)  [unwired: 1 out]
              "Input Voltage _V_" <- w179
              "Phase Input Voltage _deg_" <- w180
            }
            frame "HW (Uhw)" {
              w199 = T9 1 items=["Trapezoidal Rule", "Simpson's Rule", "Simpson's 3/8 Rule", "Bode Rule"] ("integration method")
              n72 = Reciprocal(x=w198) -> (1/x=w197:dbl)
              n73 = local read "Frequency (Hz)"() -> (w193:dbl)
              n74 = local read "nu"() -> (w187:dbl)
              n75 = local read "Omega"() -> (w188:dbl)
              n76 = call-poly <vilib>:"Numeric Integration.vi"("integration method"=w199, "dt"=w197, "Input Array"=w200) -> ("result"=w196:dbl)  [unwired: 1 out]
              n77 = Subtract(x=w202, y=w203) -> (x-y=→"Phase Velocity _deg_":dbl)
              n78 = Square(x=w189) -> (x^2=w190:dbl)
              n79 = Divide(x=w196, y=2.0) -> (x/y=w194:dbl)
              "Stroke Length _m_" <- w194
              n80 = Multiply(x=w188, y=w190) -> (x*y=w186:dbl)
              n81 = Multiply(x=w193, y=w194) -> (x*y=w192:dbl)
              "Charicteristic Velocity m_s" <- w192
              n82 = Multiply(x=w192, y=w189) -> (x*y=w191:dbl)
              n83 = Divide(x=w191, y=w187) -> (x/y=w184:dbl)
              "Reynolds Number" <- w184
              n84 = Divide(x=w186, y=w187) -> (x/y=w185:dbl)
              n85 = Square Root(x=w185) -> (sqrt(x)=w182:dbl)
              "Stokes Number" <- w182
              n86 = Square(x=w182) -> (x^2=w183:dbl)
              n87 = Divide(x=w183, y=w184) -> (x/y=→"Strouhal Number":dbl)
              "Velocity m_s" <- w200
              "RMS Velocity m_s" <- w205
              "Max Velocity m_s" <- w204
            }
            frame "RV (Vdi)" {
              n88 = Subtract(x=w206, y=w207) -> (x-y=→"Phase Displ _deg_":dbl)
              "Displacement _m_" <- w211
              "Max Displacement _m_" <- w209
              "RMS Dispacement _m_" <- w210
            }
            frame "Mano (Pressure)" {
              n89 = Subtract(x=w214, y=w213) -> (x-y=→"Phase Pressure _deg_":dbl)
              "Pressure _Pa_" <- w217
              "RMS Pressure _Pa_" <- w216
              "Max Pressure _Pa_" <- w215
            }
            frame "RV (Pressure)" {
              n90 = Subtract(x=w220, y=w219) -> (x-y=→"RV Phase Pressure _deg_":dbl)
              "RV Pressure _V_" <- w223
              "RV Max Pressure _V_" <- w221
              "RV RMS Pressure _V_" <- w222
            }
            frame "Pitot (Pitot)" {
            }
            frame "RV (Current)" {
              n91 = local read "Frequency (Hz)"() -> (w225:dbl)
              n92 = Multiply(x=w240, y=w239) -> (x*y=w238:dbl[])
              n93 = Reciprocal(x=w229) -> (1/x=w228:dbl)
              n94 = Multiply(x=w245, y=w246) -> (x*y=w227:dbl[])
              "Power_W_" <- w227
              n95 = call "SJ_Get_Signal_Phase.vi"("No of Analogue Samples"=w235, "Number of Cycles"=w236, "Actual Sampling Frequency"=w237, "Signal"=w238) -> ("Phase Angle"=w234:dbl)  [unwired: 7 in]
              n96 = Subtract(x=w230, y=w232) -> (x-y=→"Phase Current _deg_":dbl)
              n97 = Subtract(x=w230, y=w234) -> (x-y=→"Phase Power _deg_":dbl)
              n98 = call-poly <vilib>:"RMS.vi"("X"=w227) -> ("rms value"=→"RMS Power _W_":dbl)  [unwired: 1 out]
              n99 = Array Max & Min(array=w227) -> (max value=→"Max Power _W_":dbl)  [unwired: 3 out]
              n100 = call-poly <vilib>:"Numeric Integration.vi"("dt"=w228, "Input Array"=w227) -> ("result"=w226:dbl)  [unwired: 1 in, 1 out]
              n101 = Multiply(x=w226, y=w225) -> (x*y=→"Int Power _W_":dbl)
              "Current _A_" <- w245
              "RMS Current _A_" <- w243
              "Max Current _A_" <- w242
            }
            frame "No Match", Default {
              n102 = One Button Dialog(message="Error in Signal Analysis", button name ("OK")="STOP") -> (true=w248:bool)
              n103 = Stop(stop? (T)=w248) -> ()
            }
          }
        }
        n104 = Divide(x=w129, y=w120) -> (x/y=w122:dbl)
        n105 = Divide(x=w124, y=w120) -> (x/y=w121:dbl)
        n106 = Subtract(x=w132, y=0.006) -> (x-y=w130:dbl)
        n107 = Subtract(x=w122, y=w130) -> (x-y=w128:dbl)
        n108 = Divide(x=w119, y=2.0) -> (x/y=w125:dbl)
        n109 = Divide(x=w128, y=w119) -> (x/y=→"DL:Streamwise:Position":dbl)
        n110 = Divide(x=w121, y=w125) -> (x/y=→"DL:Radius":dbl)
      }
      frame "LEM Calculations" {
        w258 = 0.5 ("value")
        n111 = local read "Strouhal Number"() -> (w268:dbl)
        n112 = local read "Charicteristic Velocity m_s"() -> (w263:dbl)
        n113 = local read "RMS Input Voltage _V_"() -> (w251:dbl)
        n114 = local read "RMS Current _A_"() -> (w252:dbl)
        n115 = Unbundle By Name(w260) -> ("Do"=w259:dbl)
        n116 = Reciprocal(x=w268) -> (1/x=w267:dbl)
        "Formation Criteria" <- w267
        n117 = local read "Int Power _W_"() -> (w254:dbl)
        n118 = Multiply(x=w252, y=w251) -> (x*y=→"RMS Power 2 _W_":dbl)
        n119 = Power Of X(1:w263, 2:3.0 ("y")) -> (0:w264:dbl)
        n120 = Greater?(x=w267, y=0.16) -> (0:→"Jet Formation":bool)
        n121 = Compound Arithmetic op=MULTIPLY(w259, w258) -> (w257:dbl)
        n122 = call "Read_Chan_Value_Gen.vi"("Desired Ch Names"=string[] ["Froude:NPL:Atmos_Press", "Aero_Tunnel:SmAD:Temp"], "Raw data file"=w271) -> ("Values"=w269:string[])  [unwired: 9 in]
        n123 = call-poly "Circle_Area_Poly.vi"("Radius"=w257) -> ("Area"=w256:dbl)  [unwired: 4 in]
        n124 = local read "Phase Pressure _deg_"() -> (w280:dbl)
        n125 = local read "Max Pressure _Pa_"() -> (w281:dbl)
        n126 = Fract/Exp String To Number(string=w269) -> (number=w289:dbl[])  [unwired: 3 in, 1 out]
        n127 = Compound Arithmetic op=MULTIPLY(w264, w258, 1.205 ("value"), w256) -> (w255:dbl)
        n128 = local read "Frequency (Hz)"() -> (w279:dbl)
        n129 = local read "Samps per cyle"() -> (w278:i32)
        n130 = Index Array(array=w289) -> (element #1=w286:dbl, element #2=w288:dbl)  [unwired: 2 in]
        n131 = Divide(x=w255, y=w254) -> (x/y=→"Jet Efficiency":dbl)
        n132 = Multiply(x=100.0 ("y"), y=w286) -> (x*y=w284:dbl)
        n133 = Add(x=w288, y=273.0) -> (x+y=w287:dbl)
        n134 = Bundle By Name(cluster=T8 {"R"=8.31451, "Mair"=0.0289645, "T"=293.0, "Patmos"=101325.0, "gamma"=1.4} ("Fluid Properties"), "Patmos"=w284, "T"=w287) -> (w282:T8)
        n135 = call "Get_LEM_Response.vi"("Frequency (Hz)"=w279, "Cavity Pressure Magnitude"=w281, "Cavity Pressure Phase"=w280, "Fluid Properties"=w282, "SJ Data IN"=w260) -> ("Phi"=w277:dbl, "Uo"=w276:dbl, "OmegaH"=w274:dbl)  [unwired: 2 in, 2 out]
        "LEM Phase Velocity _deg_" <- w277
        "LEM Max Velocity _ms_" <- w276
        n136 = call <vilib>:"Sine Pattern.vi"("phase(degrees)"=w277, "amplitude"=w276, "samples"=w278) -> ("Sinusoidal Pattern"=→"LEM Velocity _ms_":dbl[])  [unwired: 1 in, 1 out]
        n137 = Divide(x=w274, y=6.283185307179586) -> (x/y=→"Cavity:Helmholtz:Hz":dbl)
      }
      frame "Collect Mean Data" {
        n138 = local read "Samps per cyle"() -> (w360:i32)
        n139 = local read "RMS Dispacement _m_"() -> (w301:dbl)
        n140 = local read "Max Displacement _m_"() -> (w302:dbl)
        n141 = local read "Phase Current _deg_"() -> (w367:dbl)
        n142 = local read "Phase Power _deg_"() -> (w339:dbl)
        n143 = local read "Phase Pressure _deg_"() -> (w364:dbl)
        n144 = local read "Phase Displ _deg_"() -> (w300:dbl)
        n145 = local read "Int Power _W_"() -> (w361:dbl)
        n146 = local read "RMS Pressure _Pa_"() -> (w357:dbl)
        n147 = local read "Max Pressure _Pa_"() -> (w307:dbl)
        n148 = local read "RMS Current _A_"() -> (w366:dbl)
        n149 = local read "RMS Power 2 _W_"() -> (w370:dbl)
        n150 = local read "Max Power _W_"() -> (w368:dbl)
        n151 = local read "RMS Power _W_"() -> (w369:dbl)
        n152 = local read "Max Current _A_"() -> (w365:dbl)
        n153 = call-poly <vilib>:"Ramp Pattern.vi"("exclude end?"=TRUE, "start"=0.0, "end"=360.0, "samples"=w360) -> ("Ramp Pattern"=w317:dbl[])  [unwired: 6 in, 1 out]
        "Phase Angle _deg_" <- w317
        n154 = local read "LEM Velocity _ms_"() -> (w313:dbl[])
        n155 = local read "Input Voltage _V_"() -> (w348:dbl[])
        n156 = local read "Displacement _m_"() -> (w341:dbl[])
        n157 = local read "Velocity m_s"() -> (w310:dbl[])
        n158 = local read "Pressure _Pa_"() -> (w346:dbl[])
        n159 = call "Get_Variable_Name.vi"("Data"=w300) -> ("Data Name(s)"=w294:string[], "Data Values(s)"=w297:string[])  [unwired: 24 in, 1 out]
        n160 = call "Get_Variable_Name.vi"("Data"=w339) -> ("Data Name(s)"=w338:string[], "Data Values(s)"=w319:string[])  [unwired: 24 in, 1 out]
        n161 = call "Get_Variable_Name.vi"("Data"=w301) -> ("Data Name(s)"=w295:string[], "Data Values(s)"=w298:string[])  [unwired: 24 in, 1 out]
        n162 = call "Get_Variable_Name.vi"("Data"=w307) -> ("Data Name(s)"=w306:string[], "Data Values(s)"=w305:string[])  [unwired: 24 in, 1 out]
        n163 = call "Get_Variable_Name.vi"("Data"=w357) -> ("Data Name(s)"=w329:string[], "Data Values(s)"=w328:string[])  [unwired: 24 in, 1 out]
        n164 = call "Get_Variable_Name.vi"("Data"=w364) -> ("Data Name(s)"=w330:string[], "Data Values(s)"=w327:string[])  [unwired: 24 in, 1 out]
        n165 = call "Get_Variable_Name.vi"("Data"=w365) -> ("Data Name(s)"=w331:string[], "Data Values(s)"=w326:string[])  [unwired: 24 in, 1 out]
        n166 = call "Get_Variable_Name.vi"("Data"=w366) -> ("Data Name(s)"=w332:string[], "Data Values(s)"=w325:string[])  [unwired: 24 in, 1 out]
        n167 = call "Get_Variable_Name.vi"("Data"=w367) -> ("Data Name(s)"=w333:string[], "Data Values(s)"=w324:string[])  [unwired: 24 in, 1 out]
        n168 = call "Get_Variable_Name.vi"("Data"=w368) -> ("Data Name(s)"=w334:string[], "Data Values(s)"=w323:string[])  [unwired: 24 in, 1 out]
        n169 = call "Get_Variable_Name.vi"("Data"=w369) -> ("Data Name(s)"=w335:string[], "Data Values(s)"=w322:string[])  [unwired: 24 in, 1 out]
        n170 = call "Get_Variable_Name.vi"("Data"=w370) -> ("Data Name(s)"=w336:string[], "Data Values(s)"=w321:string[])  [unwired: 24 in, 1 out]
        n171 = call "Get_Variable_Name.vi"("Data"=w361) -> ("Data Name(s)"=w337:string[], "Data Values(s)"=w320:string[])  [unwired: 24 in, 1 out]
        n172 = call "Get_Variable_Name.vi"("Data"=w302) -> ("Data Name(s)"=w296:string[], "Data Values(s)"=w299:string[])  [unwired: 24 in, 1 out]
        n173 = local read "Current _A_"() -> (w343:dbl[])
        n174 = local read "Cavity:Helmholtz:Hz"() -> (w308:dbl)
        n175 = local read "Frequency (Hz)"() -> (w304:dbl)
        n176 = Build Array(w305, w328, w327, w326, w325, w324, w323, w322, w321, w320, w319, w299, w298, w297) -> (w356:string[][])
        n177 = call-poly <vilib>:"Quick Scale.vi"("X"=w313) -> ("Y[i]=X[i]/Max|X|"=w311:dbl[], "max|X|"=w312:dbl)  [unwired: 1 out]
        n178 = call-poly <vilib>:"Quick Scale.vi"("X"=w348) -> ("Y[i]=X[i]/Max|X|"=w347:dbl[])  [unwired: 2 out]
        n179 = call-poly <vilib>:"Quick Scale.vi"("X"=w346) -> ("Y[i]=X[i]/Max|X|"=w345:dbl[])  [unwired: 2 out]
        n180 = call-poly <vilib>:"Quick Scale.vi"("X"=w341) -> ("Y[i]=X[i]/Max|X|"=w344:dbl[])  [unwired: 2 out]
        n181 = call-poly <vilib>:"Quick Scale.vi"("X"=w343) -> ("Y[i]=X[i]/Max|X|"=w342:dbl[])  [unwired: 2 out]
        n182 = Build Array(w306, w329, w330, w331, w332, w333, w334, w335, w336, w337, w338, w296, w295, w294) -> (w318:string[][])
        n183 = Divide(x=w310, y=w312) -> (x/y=w309:dbl[])
        n184 = local read "Amplitude (V)"() -> (w372:dbl)
        n185 = for {
          tunnel: w356 -> [w392] mode=indexing
          tunnel: [w390] -> w353 mode=indexing
          n186 = Index Array(array=w392) -> (element=w391:string)  [unwired: 1 in]
          n187 = Fract/Exp String To Number(string=w391) -> (number=w390:dbl)  [unwired: 3 in, 1 out]
        }
        n188 = Bundle("Ramp Pattern"=w317, "Y[i]=X[i]/Max|X|"=w347) -> (w375:T10)  [unwired: 1 in]
        n189 = Bundle("Ramp Pattern"=w317, "Y[i]=X[i]/Max|X|"=w345) -> (w384:T10)  [unwired: 1 in]
        n190 = Bundle("Ramp Pattern"=w317, "Y[i]=X[i]/Max|X|"=w344) -> (w385:T10)  [unwired: 1 in]
        n191 = Bundle("Ramp Pattern"=w317, "Y[i]=X[i]/Max|X|"=w342) -> (w374:T10)  [unwired: 1 in]
        n192 = Bundle("Ramp Pattern"=w317, w309) -> (w386:cluster{"Ramp Pattern":dbl[], dbl[]})  [unwired: 1 in]
        n193 = Bundle("Ramp Pattern"=w317, "Y[i]=X[i]/Max|X|"=w311) -> (w340:T10)  [unwired: 1 in]
        n194 = for {
          tunnel: w318 -> [w389] mode=indexing
          tunnel: [w388] -> w315 mode=indexing
          n195 = Index Array(array=w389) -> (element=w388:string)  [unwired: 1 in]
        }
        "Output Data Names" <- w315
        n196 = Divide(x=w304, y=w308) -> (x/y=→"DL:Frequency":dbl)
        n197 = Build Array(w375, w384) -> (→"Pressure Plot":T11)
        n198 = Build Array(w375, w385) -> (→"Displacement Plot":T11)
        n199 = Build Array(w375, w374) -> (→"Current Plot":T11)
        n200 = Build Array(w375, w386, w340) -> (→"Velocity Plot":T11)
        n201 = Build Array(w304, w372) -> (w352:dbl[])
        n202 = property on="Menu Ring" class="Ring (strict)"("Strings []"=w315) -> ()  [unwired: 2 in, 2 out]
        n203 = Index Array(array=w315, index=w354) -> (element=w363:string)
        n204 = Insert Into Array(array=w353, index=0, new element=w352) -> (w351:dbl[])
        n205 = property on="Pressure v Frequency" class="XYGraph (strict)"("YScale.NameLbl.Text"=w363) -> ()  [unwired: 2 in, 2 out]
        n206 = Add(x=u16 2, y=w354) -> (x+y=w362:u16)
        n207 = Build Array (concatenate)(w380, w351) -> (w379:dbl[][])
        n208 = Index Array(array=w379, index (col) #1=0 ("disabled index (col)"), index (col) #2=w362) -> (element #1=w377:dbl[], element #2=w371:dbl[])  [unwired: 2 in]
        n209 = Bundle(w377, w371) -> (→"Pressure v Frequency":cluster{dbl[], dbl[]})  [unwired: 1 in]
      }
      frame "Save Phase Average File" {
        w461 = 0 ("No of Bins")
        n210 = local read "Phase Angle _deg_"() -> (w452:dbl[])
        n211 = local read "LEM Velocity _ms_"() -> (w420:dbl[])
        n212 = local read "Input Voltage _V_"() -> (w484:dbl[])
        n213 = local read "Displacement _m_"() -> (w483:dbl[])
        n214 = local read "DL:Streamwise:Position"() -> (w406:dbl)
        n215 = local read "LEM Max Velocity _ms_"() -> (w416:dbl)
        n216 = Strip Path(path=w468) -> (stripped path=w472:path)  [unwired: 1 out]
        n217 = local read "Pressure _Pa_"() -> (w480:dbl[])
        n218 = local read "Cavity:Helmholtz:Hz"() -> (w399:dbl)
        n219 = local read "Max Pressure _Pa_"() -> (w464:dbl)
        n220 = local read "Current _A_"() -> (w482:dbl[])
        n221 = local read "Velocity m_s"() -> (w479:dbl[])
        n222 = local read "Max Velocity m_s"() -> (w417:dbl)
        n223 = local read "Power_W_"() -> (w481:dbl[])
        n224 = local read "Frequency (Hz)"() -> (w398:dbl)
        n225 = local read "DL:Frequency"() -> (w466:dbl)
        n226 = local read "Amplitude (V)"() -> (w465:dbl)
        n227 = Strip Path(path=w472) -> (stripped path=w474:path, name=w477:string)
        n228 = local read "DL:Radius"() -> (w407:dbl)
        n229 = Strip Path(path=w474) -> (stripped path=w473:path)  [unwired: 1 out]
        n230 = Concatenate Strings(w477, "_" ("string"), w410, ".xls" ("string")) -> (w478:string)
        n231 = Strip Path(path=w473) -> (stripped path=w475:path)  [unwired: 1 out]
        n232 = call "Get_Variable_Name.vi"("Data"=w452) -> ("Data Name(s)"=w436:string[], "Data Values(s)"=w423:string[])  [unwired: 24 in, 1 out]
        n233 = call "Get_Variable_Name.vi"("Data"=w420) -> ("Data Name(s)"=w419:string[], "Data Values(s)"=w418:string[])  [unwired: 24 in, 1 out]
        n234 = call "Get_Variable_Name.vi"("Data"=w484) -> ("Data Name(s)"=w441:string[], "Data Values(s)"=w431:string[])  [unwired: 24 in, 1 out]
        n235 = call "Get_Variable_Name.vi"("Data"=w483) -> ("Data Name(s)"=w440:string[], "Data Values(s)"=w430:string[])  [unwired: 24 in, 1 out]
        n236 = call "Get_Variable_Name.vi"("Data"=w482) -> ("Data Name(s)"=w439:string[], "Data Values(s)"=w429:string[])  [unwired: 24 in, 1 out]
        n237 = call "Get_Variable_Name.vi"("Data"=w481) -> ("Data Name(s)"=w438:string[], "Data Values(s)"=w428:string[])  [unwired: 24 in, 1 out]
        n238 = call "Get_Variable_Name.vi"("Data"=w480) -> ("Data Name(s)"=w426:string[], "Data Values(s)"=w425:string[])  [unwired: 24 in, 1 out]
        n239 = call "Get_Variable_Name.vi"("Data"=w479) -> ("Data Name(s)"=w437:string[], "Data Values(s)"=w427:string[])  [unwired: 24 in, 1 out]
        n240 = call "Get_Variable_Name.vi"("Data"=w410) -> ("Data Name(s)"=w451:string[], "Data Values(s)"=w445:string[])  [unwired: 24 in, 1 out]
        n241 = call "Get_Variable_Name.vi"("Data"=w466) -> ("Data Name(s)"=w450:string[], "Data Values(s)"=w444:string[])  [unwired: 24 in, 1 out]
        n242 = call "Get_Variable_Name.vi"("Data"=w465) -> ("Data Name(s)"=w449:string[], "Data Values(s)"=w443:string[])  [unwired: 24 in, 1 out]
        n243 = call "Get_Variable_Name.vi"("Data"=w464) -> ("Data Name(s)"=w448:string[], "Data Values(s)"=w442:string[])  [unwired: 24 in, 1 out]
        n244 = call "Get_Variable_Name.vi"("Data"=w417) -> ("Data Name(s)"=w415:string[], "Data Values(s)"=w413:string[])  [unwired: 24 in, 1 out]
        n245 = call "Get_Variable_Name.vi"("Data"=w416) -> ("Data Name(s)"=w414:string[], "Data Values(s)"=w412:string[])  [unwired: 24 in, 1 out]
        n246 = call "Get_Variable_Name.vi"("Data"=w406) -> ("Data Name(s)"=w403:string[], "Data Values(s)"=w405:string[])  [unwired: 24 in, 1 out]
        n247 = call "Get_Variable_Name.vi"("Data"=w407) -> ("Data Name(s)"=w402:string[], "Data Values(s)"=w404:string[])  [unwired: 24 in, 1 out]
        n248 = call "Get_Variable_Name.vi"("Data"=w399) -> ("Data Name(s)"=w401:string[], "Data Values(s)"=w400:string[])  [unwired: 24 in, 1 out]
        n249 = call "Get_Variable_Name.vi"("Data"=w398) -> ("Data Name(s)"=w397:string[], "Data Values(s)"=w396:string[])  [unwired: 24 in, 1 out]
        n250 = Build Path(base path=w475, name or relative path="Results_Post_Processed") -> (appended path=w471:path)
        n251 = Build Path(base path=w471, name or relative path="Phase_Averaged" ("New Results Folder Name")) -> (appended path=w470:path)
        n252 = Build Array(w441, w440, w439, w438, w426, w437, w419) -> (w433:string[][])
        n253 = Build Path(base path=w470, name or relative path=w478) -> (appended path=w455:path)
        n254 = local read "Samps per cyle"() -> (w453:i32)
        n255 = for {
          tunnel: w433 -> [w486] mode=indexing
          tunnel: [w485] -> w432 mode=indexing
          n256 = Index Array(array=w486) -> (element=w485:string)  [unwired: 1 in]
        }
        n257 = Build Array(w431, w430, w429, w428, w425, w427, w418) -> (w424:string[][])
        n258 = call <vilib>:"Check if File or Folder Exists.vi"("path"=w455) -> ("file or folder exists?"=w393:bool, "dup path"=w394:path)  [unwired: 8 in, 1 out]
        n259 = Build Array(w451, w450, w449, w448, w415, w414, w403, w402, w401, w397) -> (w447:string[][])
        n260 = Array Size(array=w432) -> (size(s)=w454:i32)
        n261 = Build Array(w445, w444, w443, w442, w413, w412, w405, w404, w400, w396) -> (w463:string[][])
        n262 = Index Array(array=w436) -> (element=w435:string)  [unwired: 1 in]
        n263 = Compound Arithmetic op=MULTIPLY(w453, w454) -> (w434:i32)
        n264 = for {
          tunnel: w447 -> [w488] mode=indexing
          tunnel: [w487] -> w446 mode=indexing
          n265 = Index Array(array=w488) -> (element=w487:string)  [unwired: 1 in]
        }
        n266 = for {
          tunnel: w463 -> [w490] mode=indexing
          tunnel: [w489] -> w460 mode=indexing
          n267 = Index Array(array=w490) -> (element=w489:string)  [unwired: 1 in]
        }
        n268 = for {
          N: w434 -> [_]
          tunnel: w432 -> [w502]
          shift-right: [w505] -> _
          shift-left: w461 -> [w498]
          tunnel: w453 -> [w506]
          tunnel: w423 -> [w500]
          tunnel: [w491] -> w462 mode=indexing
          tunnel: w424 -> [w501]
          shift-right: [w499] -> _
          shift-left: w461 -> [w497]
          tunnel: [w496] -> w459 mode=indexing
          tunnel: w435 -> [w494]
          w493 = ":"
          n269 = Index Array(array=w502, index=w497) -> (element=w495:string)
          n270 = Index Array(array=w501, index (row)=w497, index (col)=w498) -> (element=w496:string)
          n271 = Index Array(array=w500, index=w498) -> (element=w492:string)
          n272 = Increment(x=w498) -> (x+1=w504:i32)
          n273 = Concatenate Strings(w495, w493, w494, w493, w492) -> (w491:string)
          n274 = Equal?(x=w506, y=w504) -> (x = y?=w503:bool)
          n275 = case shown="True" w503 {
            tunnel: [w508 0] -> w505
            tunnel: w504 -> [w508 _]
            tunnel: w497 -> [w507 w510]
            tunnel: [w507 w509] -> w499
            frame False {
            }
            frame True {
              n276 = Increment(x=w510) -> (x+1=w509:i32)
            }
          }
        }
        n277 = Insert Into Array(array=w460, new element=w459) -> (w456:string[])  [unwired: 1 in]
        n278 = Insert Into Array(array=w446, new element=w462) -> (w458:string[])  [unwired: 1 in]
        n279 = Build Array(w456) -> (w457:string[][])
        n280 = call "Write_Ch_data_file.vi"("Append last row only"=FALSE, "exists?"=w393, "Channel Values"=w457, "Channel names"=w458, "Filename"=w394) -> ()  [unwired: 7 in]
      }
      frame "Save Mean Data" {
        n281 = local read "Output Data Names"() -> (w561:string[])
        n282 = Build Array("Aero_Tunnel:Abs Pressure:Bar" ("element")) -> (w514:string[])
        n283 = Array Subset(array=w558, index (col)=2 ("index")) -> (w562:dbl[][])  [unwired: 3 in]
        n284 = call "Read_Chan_Value_Gen.vi"("Desired Ch Names"=w514, "Raw data file"=w516) -> ("Values"=w513:string[])  [unwired: 9 in]
        n285 = local read "Disc ID"() -> (w536:i32)
        n286 = local read "Jet ID"() -> (w535:string)
        n287 = Unbundle By Name(w557) -> ("Do"=w556:dbl, "Dc"=w555:dbl, "Ho"=w554:dbl, "Hc"=w553:dbl, "K"=w552:dbl, "beta"=w551:dbl)
        n288 = Index Array(array=w513) -> (element=w512:string)  [unwired: 1 in]
        n289 = Index Array(array=w558, index (col) #1=1 ("disabled index (col)"), index (col) #2=0 ("index (col)")) -> (element #1=w540:dbl[], element #2=w539:dbl[])  [unwired: 2 in]
        n290 = Build Array(w512) -> (w529:string[])
        n291 = Build Array("Atmospheric Pressure:Pa" ("string")) -> (w530:string[])
        n292 = Build Array(w532) -> (w528:string[])
        n293 = Build Array("Comment:String" ("string")) -> (w550:string[])
        n294 = call "Get_Variable_Name.vi"("Data"=w556) -> ("Data Name(s)"=w549:string[], "Data Values(s)"=w527:string[])  [unwired: 24 in, 1 out]
        n295 = call "Get_Variable_Name.vi"("Data"=w555) -> ("Data Name(s)"=w548:string[], "Data Values(s)"=w526:string[])  [unwired: 24 in, 1 out]
        n296 = call "Get_Variable_Name.vi"("Data"=w554) -> ("Data Name(s)"=w547:string[], "Data Values(s)"=w525:string[])  [unwired: 24 in, 1 out]
        n297 = call "Get_Variable_Name.vi"("Data"=w553) -> ("Data Name(s)"=w546:string[], "Data Values(s)"=w524:string[])  [unwired: 24 in, 1 out]
        n298 = call "Get_Variable_Name.vi"("Data"=w552) -> ("Data Name(s)"=w545:string[], "Data Values(s)"=w523:string[])  [unwired: 24 in, 1 out]
        n299 = call "Get_Variable_Name.vi"("Data"=w551) -> ("Data Name(s)"=w544:string[], "Data Values(s)"=w522:string[])  [unwired: 24 in, 1 out]
        n300 = call "Get_Variable_Name.vi"("Data"=w536) -> ("Data Name(s)"=w534:string[], "Data Values(s)"=w521:string[])  [unwired: 24 in, 1 out]
        n301 = call "Get_Variable_Name.vi"("Data"=w535) -> ("Data Name(s)"=w533:string[], "Data Values(s)"=w520:string[])  [unwired: 24 in, 1 out]
        n302 = for {
          tunnel: w516 -> [w601]
          tunnel: w561 -> [w600] mode=indexing
          tunnel: [w598] -> w560 mode=indexing
          tunnel: [w597] -> w559 mode=indexing
          n303 = call "Get_New_Path_from_raw_data.vi"("New Results File Name"=w600, "New Results Folder Name"="_Mean_Data" ("string"), "Raw data file"=w601) -> ("Does it already exist?"=w598:bool, "New Spreadsheet Results File"=w597:path)  [unwired: 7 in]
        }
        n304 = for {
          tunnel: "Amp & Freq:" ("string") -> [w580]
          tunnel: w540 -> [w579] mode=indexing
          tunnel: w539 -> [w575] mode=indexing
          tunnel: [w573] -> w537 mode=indexing
          w574 = i16 3 ("precision (6)")
          n305 = Number To Fractional String(number=w579, precision (6)=w574) -> (F-format string=w578:string)  [unwired: 2 in]
          n306 = Number To Fractional String(number=w575, precision (6)=w574) -> (F-format string=w576:string)  [unwired: 2 in]
          n307 = Concatenate Strings(w580, w578, ":" ("string"), w576) -> (w573:string)
        }
        n308 = Build Array(w530, w550, w549, w548, w547, w546, w545, w544, w534, w533) -> (w543:string[][])
        n309 = Build Array(w529, w528, w527, w526, w525, w524, w523, w522, w521, w520) -> (w519:string[][])
        n310 = for {
          tunnel: w543 -> [w582] mode=indexing
          tunnel: [w581] -> w538 mode=indexing
          n311 = Index Array(array=w582) -> (element=w581:string)  [unwired: 1 in]
        }
        n312 = for {
          tunnel: w519 -> [w572] mode=indexing
          tunnel: [w571] -> w518 mode=indexing
          n313 = Index Array(array=w572) -> (element=w571:string)  [unwired: 1 in]
        }
        n314 = disable-structure shown="Disabled" {
          frame Disabled {
            n315 = call "Ch_Active_Control_Client.vi"("Match"="Synthetic_Jet", "Activate Channels?"=FALSE, "Control on"=enum16{"Channel Name", "Main Address"}."Channel Name") -> ()  [unwired: 2 out]
          }
          frame Enabled {
          }
        }
        n316 = Insert Into Array(array=w538, new element=w537) -> (w517:string[])  [unwired: 1 in]
        n317 = for {
          tunnel: w562 -> [w593]
          tunnel: w560 -> [w591] mode=indexing
          tunnel: w559 -> [w589] mode=indexing
          tunnel: w518 -> [w587]
          tunnel: w517 -> [w583]
          i -> [w592]
          n318 = Index Array(array=w593, index (col)=w592) -> (element=w588:dbl[])  [unwired: 1 in]
          n319 = for {
            tunnel: w588 -> [w596] mode=indexing
            tunnel: [w595] -> w586 mode=indexing
            n320 = Number To Fractional String(number=w596, precision (6)=i16 7) -> (F-format string=w595:string)  [unwired: 2 in]
          }
          n321 = Insert Into Array(array=w587, new element=w586) -> (w585:string[])  [unwired: 1 in]
          n322 = Build Array(w585) -> (w584:string[][])
          n323 = call "Write_Ch_data_file.vi"("Append last row only"=FALSE, "exists?"=w591, "Channel Values"=w584, "Channel names"=w583, "Filename"=w589) -> ()  [unwired: 7 in]
        }
      }
    }
  }
